vi "Get ZeroJet Directory.vi"(7 "Expect file to be present":bool, 11 "Data directory subpath":path=path "") -> (0 "error out":errorcluster, 2 "Already exists":bool, 3 "appended path":path)   [LabVIEW 2024]
uses:
  <userlib>/_OpenG.lib/file/file.llb/File Exists - Scalar__ogtk.vi
  <userlib>/_OpenG.lib/file/file.llb/openg_file.lvlib
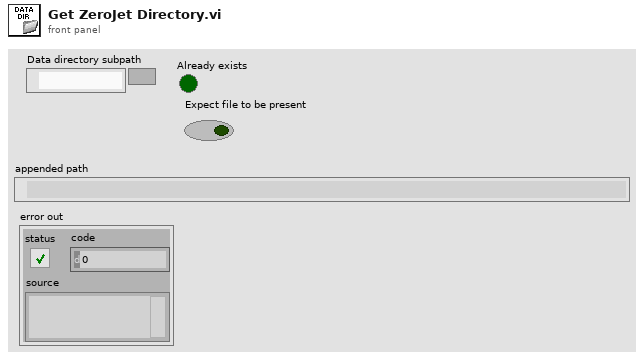
[diagram p1: front panel]
types:
  T1 = enum32{"invalid app kind", "Development System", "Run Time System", "Student Edition", "Embedded LabVIEW", "Evaluation", "Custom"}
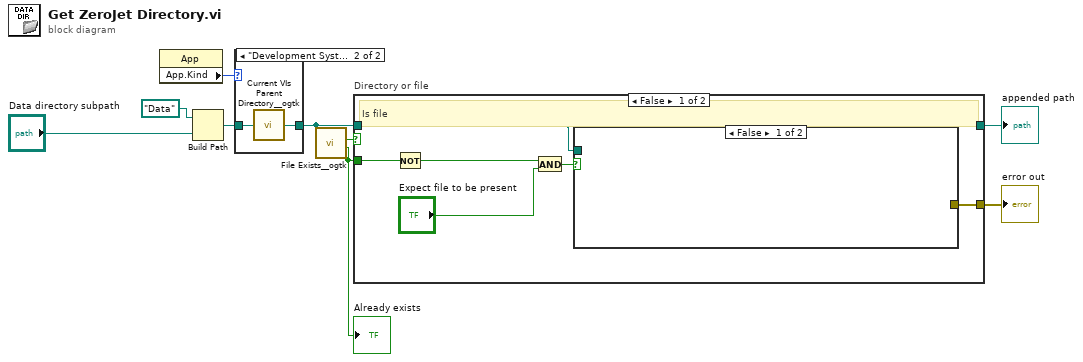
[diagram p0: block diagram]
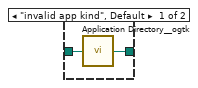
[diagram p2: hidden frame]
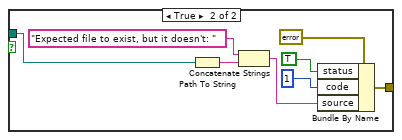
[diagram p3: hidden frame]
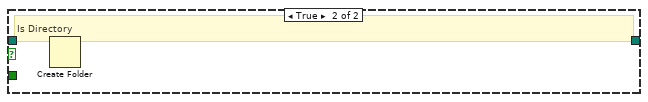
[diagram p4: hidden frame]
diagram:
  n1 = property class="App"() -> ("App.Kind"=w5:T1)  [unwired: 2 in, 2 out]
  n2 = Build Path(base path=path "Data", name or relative path="Data directory subpath") -> (appended path=w1:path)
  n3 = case shown="\"Development System\", \"Evaluation\"" w5 {
    tunnel: [w11 w12] -> w4
    tunnel: w1 -> [w10 w13]
    frame "invalid app kind", Default {
      n4 = call <userlib>:"Application Directory__ogtk.vi"("Relative path (.)"=w10) -> ("Application Directory (+ Relative)"=w11:path)
    }
    frame "Development System", "Evaluation" {
      n5 = call <userlib>:"Current VIs Parent Directory__ogtk.vi"("Relative path (.)"=w13) -> ("Parent Directory (+ Relative)"=w12:path)  [unwired: 4 in]
    }
  }
  n6 = call-poly <userlib>:"File Exists__ogtk.vi"("file path"=w4) -> ("is directory"=w8:bool, "exists"=w7:bool)  [unwired: 6 in]
  "Already exists" <- w7
  n7 = case "Directory or file" shown="False" w8 {
    tunnel: [w16 w29] -> w9
    tunnel: w4 -> [w16 w28]
    tunnel: w7 -> [w17 _]
    tunnel: [w15 _] -> w6
    frame False {
      # "Is file"
      n8 = Not(x=w17) -> (.not. x?=w14:bool)
      n9 = And(x=w14, y="Expect file to be present") -> (x .and. y?=w19:bool)
      n10 = case shown="False" w19 {
        tunnel: w16 -> [_ w24]
        tunnel: [_ w20] -> w15
        frame False {
        }
        frame True {
          n11 = Path To String(path=w24) -> (string=w22:string)
          n12 = Concatenate Strings("Expected file to exist, but it doesn't: " ("string"), w22) -> (w21:string)
          n13 = Bundle By Name(cluster=errorcluster {"status"=FALSE, "code"=0, "source"=""} ("error in (no error)"), "status"=TRUE, "code"=1, "source"=w21) -> (w20:errorcluster)
        }
      }
    }
    frame True {
      # "Is Directory"
      n14 = Create Folder(path (use dialog)=w28) -> (created path=w29:path)  [unwired: 2 in, 2 out]
    }
  }
  "appended path" <- w9
  "error out" <- w6
